vi "RT Init.vi"(8 "error in":errorcluster, 11 "Device Ref":T5=18446744073709551615 format="%.0x") -> (0 "error out":errorcluster, 3 "RT Data":T1 {"StatusRefs" format="%.0x"; "ReceiveRefs"."Data Reference" format="%.0x"; "SendRefs"."Data Reference" format="%.0x"})   [LabVIEW 2016, in "PXImc Engine.lvlib"]
uses:
  PXImc Engine.lvlib
  <vilib>/NI Veristand/Custom Device API/Custom Device Item Ref.ctl
  RT Data Cluster.ctl
  Shared/Compiled Data.ctl
  <vilib>/NI Veristand/Custom Device API/Block Data Reference.ctl
  <vilib>/NI Veristand/Custom Device API/Data Reference.ctl
  <vilib>/NI Veristand/Custom Device API/Data Access Type.ctl
  <vilib>/pximc/Initialize Reader Session (DBL).vi
  <vilib>/pximc/Initialize Writer Session (DBL).vi
  <vilib>/NI Veristand/Custom Device API/Get Item Property (Variant).vi
  Shared/Constants.vi
  <vilib>/NI Veristand/Custom Device API/Custom Device API.lvlib
  Shared/PXImc Shared.lvlib
  <vilib>/pximc/nipximc.lvlib
  <resource>/objmgr/pximc.rc
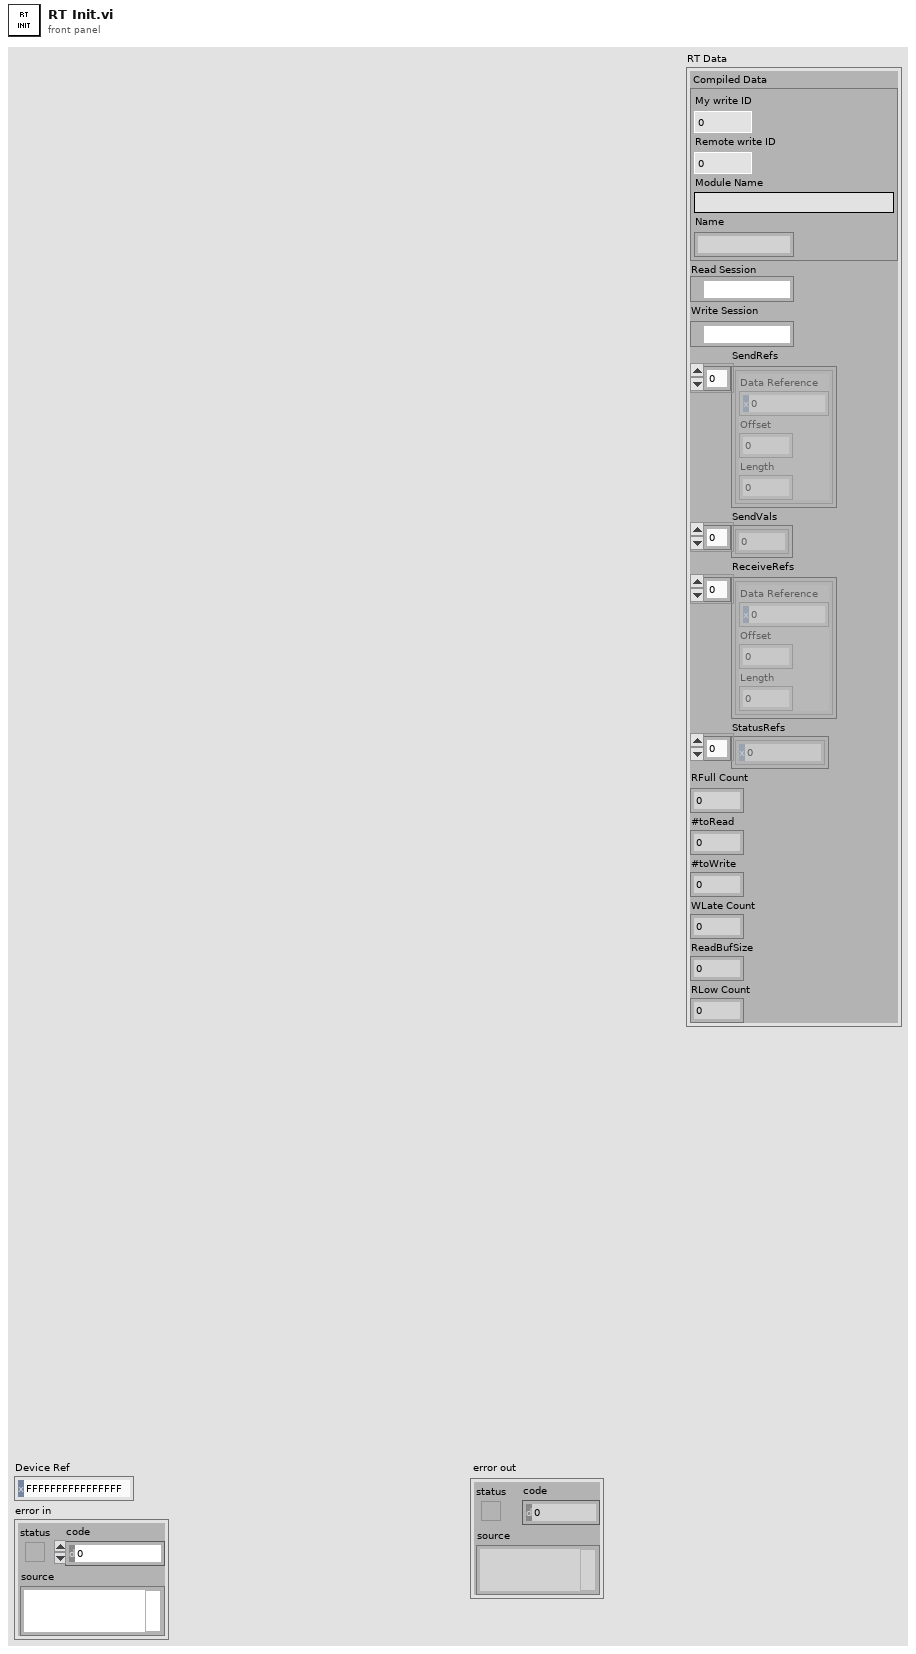
[diagram p1: front panel]
types:
  T1 = typedef "PXImc Engine.lvlib/RT Data Cluster.ctl" = cluster{"Compiled Data":T2, "Read Session":refnum<k21>, "Write Session":refnum<k21>, "SendRefs":T3[], "SendVals":dbl[], "ReceiveRefs":T3[], "StatusRefs":T4[], "RFull Count":dbl, "#toRead":i32, "#toWrite":i32, "WLate Count":dbl, "ReadBufSize":i32, "RLow Count":dbl}
  T2 = typedef "PXImc Shared.lvlib/Compiled Data.ctl" = cluster{"My write ID":u16, "Remote write ID":u16, "Module Name":string, "Name":string}
  T3 = typedef "Custom Device API.lvlib/Block Data Reference.ctl" = cluster{"Data Reference":T4, "Offset":u64, "Length":u64}
  T4 = typedef "Custom Device API.lvlib/Data Reference.ctl" = i32
  T5 = typedef "Custom Device API.lvlib/Custom Device Item Ref.ctl" = u64
  T6 = typedef "Custom Device API.lvlib/Data Access Type.ctl" = enum16{"Read", "Write"}
  T7 = typedef "PXImc Shared.lvlib/Channel.ctl" = cluster{"Name":string, "Units":string, "Default":dbl, "Description":string}
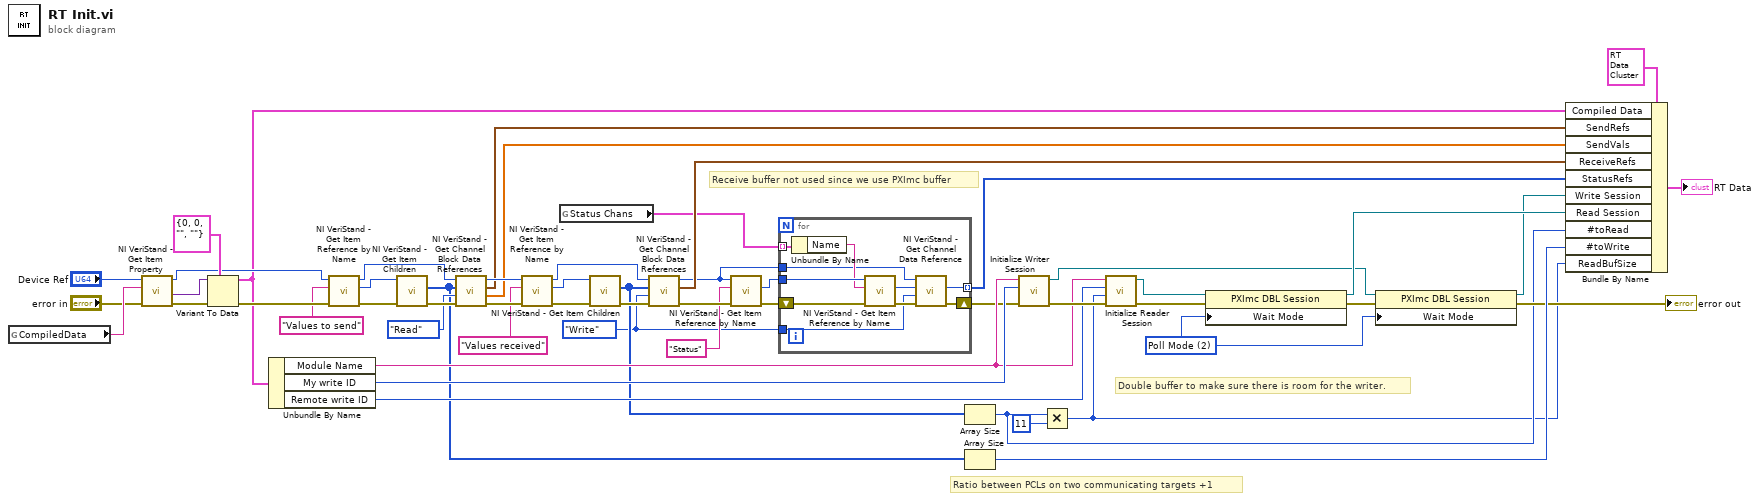
[diagram p0: block diagram]
diagram:
  w6 = u64 2 items=["Interrupt Mode"=1, "Poll Mode"=2] ("Wait Mode")
  w15 = Data_Access_Type."Write" ("Access")
  # "Ratio between PCLs on two communicating targets +1"
  # "Double buffer to make sure there is room for the writer."
  # "Receive buffer not used since we use PXImc buffer"
  n1 = global read "Constants.vi" "CompiledData"() -> (w54:string)
  n2 = call-poly <vilib>:"NI VeriStand - Get Item Property.vi"("error in (no error)"="error in", "Property Name"=w54, "Item Ref in"="Device Ref") -> ("error out"=w53:errorcluster, "Value"=w50:variant, "Item Ref out"=w45:T5)  [unwired: 5 in, 1 out]
  n3 = Variant To Data(error in=w53, type=T2 {"My write ID"=0, "Remote write ID"=0, "Module Name"="", "Name"=""} ("Compiled Data"), Variant=w50) -> (data=w26:T2, error out=w46:errorcluster)
  n4 = Unbundle By Name(w26) -> ("Module Name"=w23:string, "My write ID"=w25:u16, "Remote write ID"=w22:u16)
  n5 = call <vilib>:"NI VeriStand - Get Item Reference by Name.vi"("error in (no error)"=w46, "Item Name"="Values to send", "Parent Ref in"=w45) -> ("error out"=w43:errorcluster, "Item Ref"=w41:T5, "Parent Ref out"=w40:T5)  [unwired: 5 in, 1 out]
  n6 = call <vilib>:"NI VeriStand - Get Item Children.vi"("error in (no error)"=w43, "Item Ref in"=w41) -> ("error out"=w42:errorcluster, "Child Refs"=w12:T5[])  [unwired: 6 in, 2 out]
  n7 = call <vilib>:"NI VeriStand - Get Channel Block Data References.vi"("error in (no error)"=w42, "Access"=Data_Access_Type."Read", "Channel Refs"=w12, "Device Ref in"=w40) -> ("error out"=w34:errorcluster, "Values Array"=w30:dbl[], "Block Data Refs"=w31:T3[], "Device Ref out"=w33:T5)  [unwired: 4 in]
  n8 = call <vilib>:"NI VeriStand - Get Item Reference by Name.vi"("error in (no error)"=w34, "Item Name"="Values received", "Parent Ref in"=w33) -> ("error out"=w35:errorcluster, "Item Ref"=w37:T5, "Parent Ref out"=w38:T5)  [unwired: 5 in, 1 out]
  n9 = global read "Constants.vi" "Status Chans"() -> (w18:T7[])
  n10 = call <vilib>:"NI VeriStand - Get Item Children.vi"("error in (no error)"=w35, "Item Ref in"=w37) -> ("error out"=w36:errorcluster, "Child Refs"=w20:T5[])  [unwired: 6 in, 2 out]
  n11 = call <vilib>:"NI VeriStand - Get Channel Block Data References.vi"("error in (no error)"=w36, "Access"=w15, "Channel Refs"=w20, "Device Ref in"=w38) -> ("error out"=w28:errorcluster, "Block Data Refs"=w29:T3[], "Device Ref out"=w14:T5)  [unwired: 4 in, 1 out]
  n12 = call <vilib>:"NI VeriStand - Get Item Reference by Name.vi"("error in (no error)"=w28, "Item Name"="Status" ("New Section Name (none)"), "Parent Ref in"=w14) -> ("error out"=w19:errorcluster, "Item Ref"=w16:T5)  [unwired: 5 in, 2 out]
  n13 = for {
    shift-right: [w59] -> w17
    shift-left: w19 -> [w64]
    tunnel: w18 -> [w62] mode=indexing
    tunnel: w16 -> [w63]
    tunnel: w15 -> [w58]
    tunnel: w14 -> [w56]
    tunnel: [w55] -> w13 mode=indexing
    n14 = Unbundle By Name(w62) -> ("Name"=w61:string)
    n15 = call <vilib>:"NI VeriStand - Get Item Reference by Name.vi"("error in (no error)"=w64, "Item Name"=w61, "Parent Ref in"=w63) -> ("error out"=w60:errorcluster, "Item Ref"=w57:T5)  [unwired: 5 in, 2 out]
    n16 = call <vilib>:"NI VeriStand - Get Channel Data Reference.vi"("error in (no error)"=w60, "Access"=w58, "Channel Ref in"=w57, "Device Ref in"=w56) -> ("error out"=w59:errorcluster, "Channel Data Reference"=w55:T4)  [unwired: 5 in, 1 out]
  }
  n17 = Array Size(array=w20) -> (size(s)=w2:i32)
  n18 = Array Size(array=w12) -> (size(s)=w11:i32)
  n19 = call-poly <vilib>:"Initialize Writer Session.vi"("error in (no error)"=w17, "connection id (1)"=w25, "interface"=w23) -> ("error out"=w24:errorcluster, "session out"=w7:refnum<k21>)  [unwired: 7 in]
  n20 = Multiply(x=w2, y=11) -> (x*y=w1:i32)
  n21 = call-poly <vilib>:"Initialize Reader Session.vi"("error in (no error)"=w24, "buffer size"=w1, "writer's connection id (1)"=w22, "interface"=w23) -> ("error out"=w21:errorcluster, "session out"=w10:refnum<k21>)  [unwired: 6 in]
  n22 = property class="PXImc DBL Session"(reference=w10, error in=w21, "Wait Mode"=w6) -> (reference out=w9:refnum<k21>, error out=w8:errorcluster)
  n23 = property class="PXImc DBL Session"(reference=w7, error in=w8, "Wait Mode"=w6) -> (reference out=w4:refnum<k21>, error out=→"error out":errorcluster)
  n24 = Bundle By Name(cluster=T1 {"Compiled Data"={"My write ID"=0, "Remote write ID"=0, "Module Name"="", "Name"=""}, "Read Session"="", "Write Session"="", "SendRefs"=[], "SendVals"=[], "ReceiveRefs"=[], "StatusRefs"=[], "RFull Count"=0.0, "#toRead"=0, "#toWrite"=0, "WLate Count"=0.0, "ReadBufSize"=0, "RLow Count"=0.0}, "Compiled Data"=w26, "SendRefs"=w31, "SendVals"=w30, "ReceiveRefs"=w29, "StatusRefs"=w13, "Write Session"=w4, "Read Session"=w9, "#toRead"=w2, "#toWrite"=w11, "ReadBufSize"=w1) -> (→"RT Data":T1)
